vi "Handle Special Files.vi"(8 "error in (no error)":errorcluster, 11 "Path In":path) -> (0 "error out":errorcluster, 3 "Path Out":path)   [LabVIEW 2016, in "Folder Shot.lvlib"]
uses:
  Folder Shot.lvlib
  Source/SLL File IO/SLL File IO.lvlib
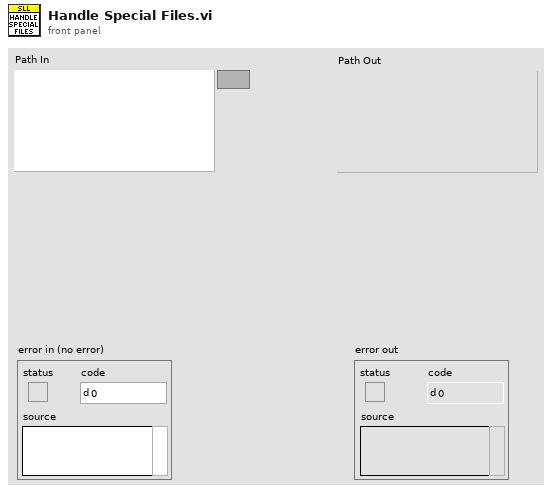
[diagram p1: front panel]
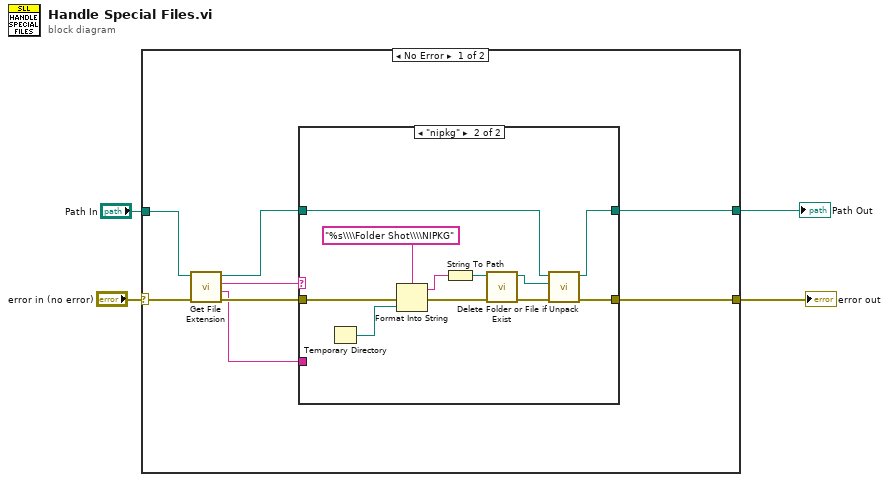
[diagram p0: block diagram]
diagram:
  n1 = case shown="No Error" "error in (no error)" {
    selector: "error in (no error)" -> [w12 w27]
    tunnel: [w9 w27] -> w3
    tunnel: "Path In" -> [w10 w26]
    tunnel: [w6 w26] -> w1
    frame No Error {
      n2 = call <vilib>:"Get File Extension.vi"("error in (no error)"=w12, "file"=w10) -> ("error out"=w11:errorcluster, "filename without extension"=w5:string, "lowercase file extension"=w8:string, "dup file"=w7:path)  [unwired: 5 in, 1 out]
      n3 = case shown="\"nipkg\"" w8 {
        tunnel: w11 -> [w13 w23]
        tunnel: [w13 w25] -> w9
        tunnel: w7 -> [w14 w24]
        tunnel: [w14 w19] -> w6
        tunnel: w5 -> [_ _]
        frame "", Default {
        }
        frame "nipkg" {
          n4 = Temporary Directory() -> (w18:path)
          n5 = Format Into String(format string="%s\\\\Folder Shot\\\\NIPKG", error in=w23, w18) -> (resulting string=w20:string, error out=w22:errorcluster)  [unwired: 1 in]
          n6 = String To Path(string=w20) -> (path=w16:path)
          n7 = call "Delete Folder or File if Exist.vi"("error in (no error)"=w22, "Path"=w16) -> ("error out"=w17:errorcluster, "Path out"=w15:path)  [unwired: 8 in]
          n8 = call <vilib>:"Unpack.vi"("error in"=w17, "destination folder"=w15, "nipkg filepath"=w24) -> ("error out"=w25:errorcluster, "unpacked folderpath"=w19:path)  [unwired: 4 in, 3 out]
        }
      }
    }
    frame Error {
    }
  }
  "error out" <- w3
  "Path Out" <- w1
